vi "Test Bench v13 - TDMS.vi"() -> ()   [LabVIEW 2022 SP3]
uses:
  WhiteNoise.ctl
  <vilib>/Utility/error.llb/DialogType.ctl
  <vilib>/DAQmx/read.llb/DAQmx Read (Analog 1D DBL 1Chan NSamp).vi
  <vilib>/DAQmx/write.llb/DAQmx Write (Analog 2D DBL NChan NSamp).vi
  <vilib>/DAQmx/create/channels.llb/DAQmx Create Channel (AI-Acceleration-Accelerometer).vi
  <vilib>/DAQmx/create/channels.llb/DAQmx Create Channel (AO-Voltage-Basic).vi
  <vilib>/DAQmx/configure/timing.llb/DAQmx Timing (Sample Clock).vi
  <vilib>/DAQmx/miscellaneous.llb/DAQmx Fill In Error Info.vi
  <resource>/objmgr/daqmx.rc
  <vilib>/measure/NI_MABase.lvlib
panel:
  in  "Enable Display":bool=TRUE
  in  "Folder to save file to":path=path "C:/Users/LAV-UFSC/OneDrive - UFSC/Documents-LAV-UFSC/LAV-TCC/Dados-Experimentos/Dados-Bancada-LABVIEW"
  out "Waveform Chart 3":dbl[](graph)
  out "Waveform Chart":dynamicdata(graph)
  in  "Accel. 2":bool
  in  "Start\nReading":bool=TRUE
  out "New file path":path
  in  "Signal Output\nControl":enum32{"White Noise", "Harmonic"}(tab)
  in  "White Noise\nParameters":T2={"Seed"=0.0, "Standard Deviation"=0.2, "Reset"=FALSE, "Iterator"=1.0, "Seed"=-1, "Stop 4"=FALSE, "Lower Cut-Off"=5.0, "Upper Cut-Off"=350.0} {"Upper Cut-Off" min=5.0 max=350.0 step=10.0; "Lower Cut-Off" min=5.0 max=350.0 step=10.0; "Standard Deviation" min=0.001 max=1.5 step=0.05 format="%0.2p"}
  out "dt White Noise":dbl
  in  "Hamonic\nParameters":T3={"Waveform Type"=0, "Frequency"=10.0, "Amplitude"=0.25, "Stop 4"=FALSE} {"Frequency" min=5.0 max=350.0 step=10.0 format="%0.2p"; "Waveform Type" items=["Sine Wave", "Triangle Wave", "Square Wave", "Sawtooth Wave"]; "Amplitude" min=0.001 max=0.3 step=0.05 format="%0.2p"}
  out "dt Harmonic":dbl
  in  "Start\nOutput":bool=TRUE
  # "Filter"
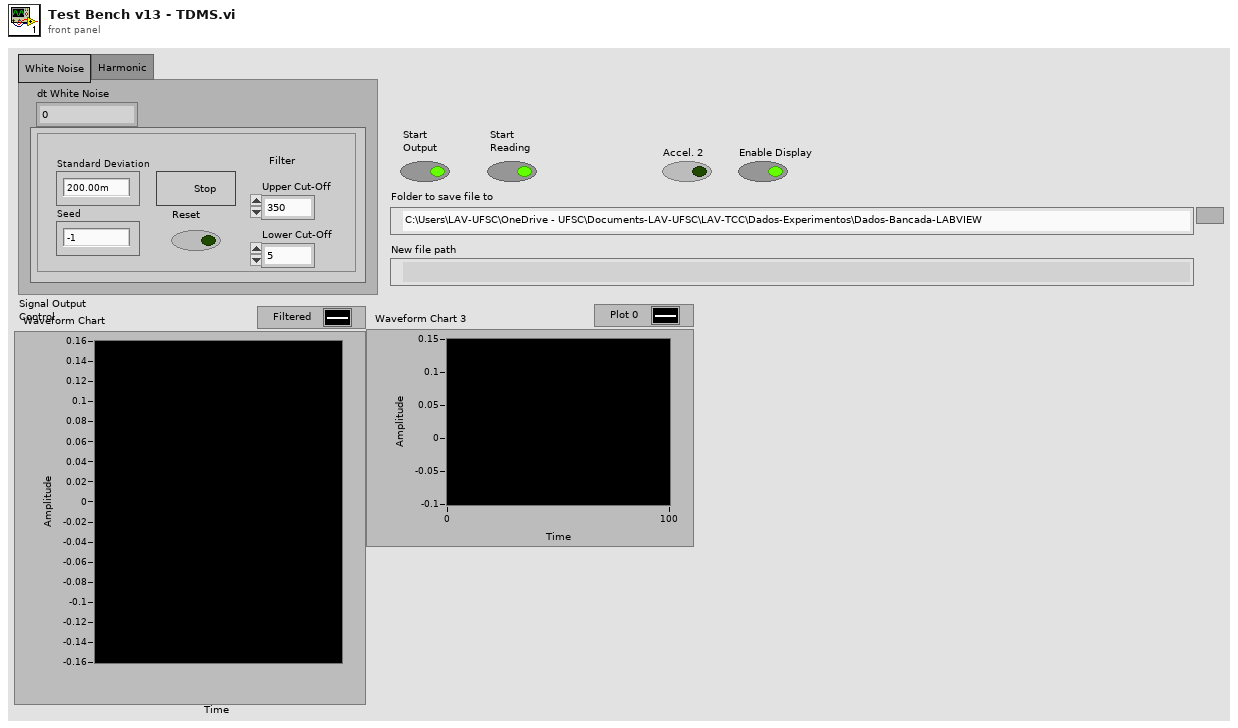
[diagram p1: front panel]
types:
  T1 = typedef "WhiteNoise.ctl" = dbl
  T2 = cluster{"Seed":T1, "Standard Deviation":dbl, "Reset":bool, "Iterator":dbl, "Seed":i8, "Stop 4":bool, "Lower Cut-Off":dbl, "Upper Cut-Off":dbl}
  T3 = cluster{"Waveform Type":u16, "Frequency":dbl, "Amplitude":dbl, "Stop 4":bool}
  T4 = enum16{"open", "open or create", "create or replace", "create", "open (read-only)"}
  T5 = typedef "DialogType.ctl" = u16
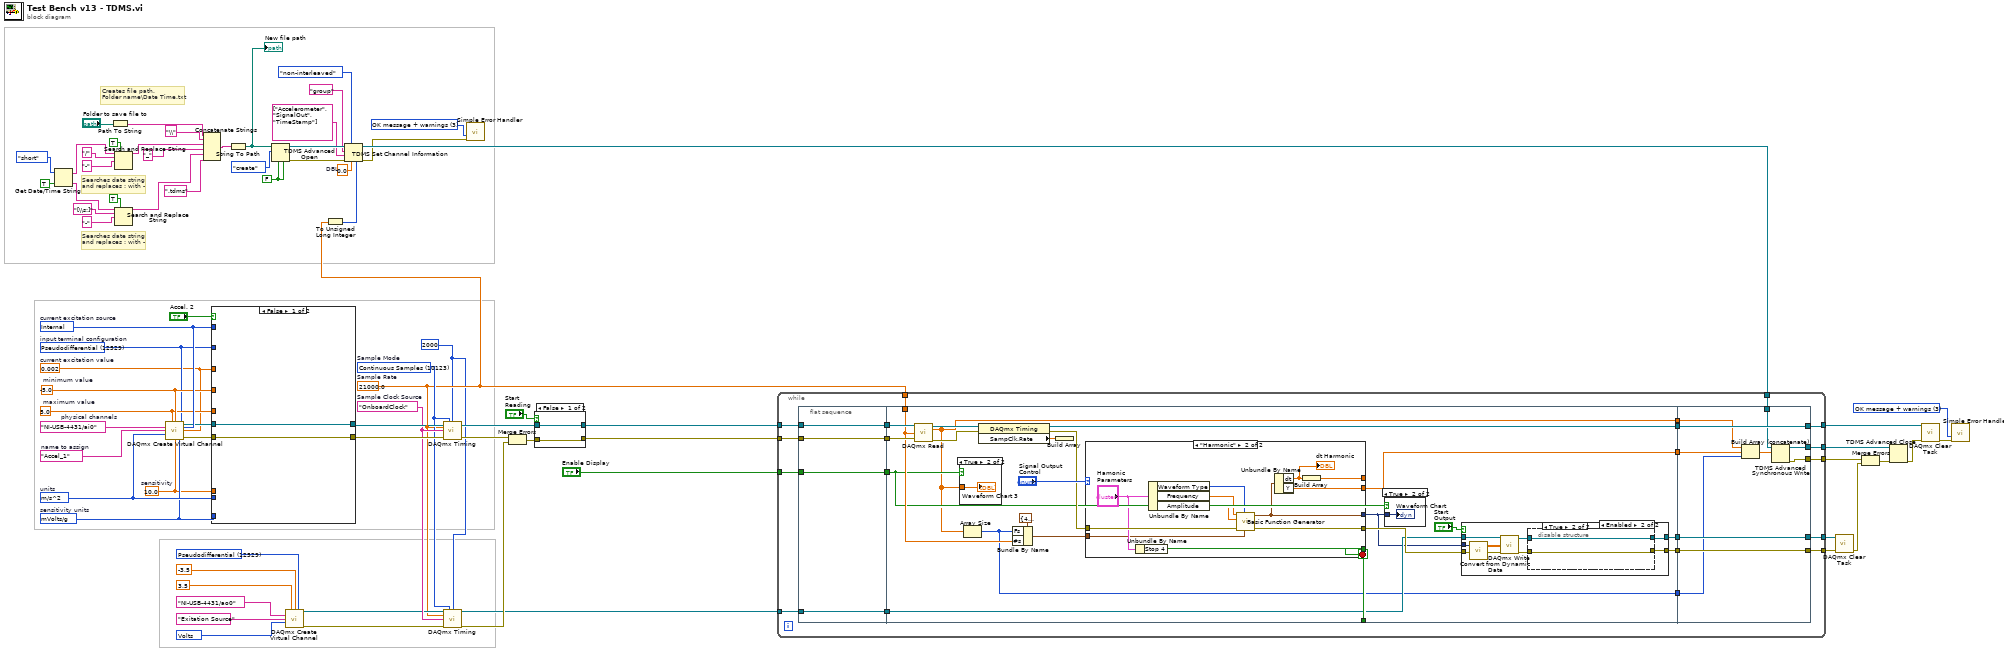
[diagram p0: block diagram]
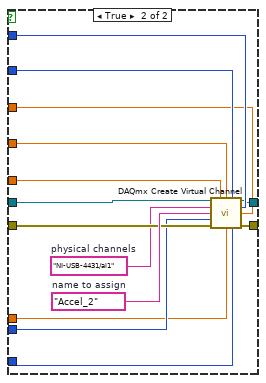
[diagram p2: hidden frame]
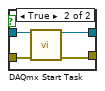
[diagram p3: hidden frame]
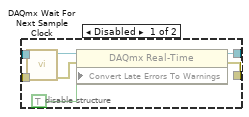
[diagram p7: hidden frame]
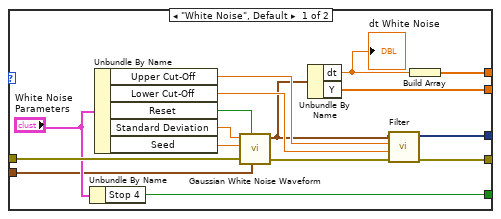
[diagram p8: hidden frame]
diagram:
  w1 = 2000 ("samples per channel")
  w9 = 0.0  # DBL
  w11 = FALSE ("enable asynchronous? (T)")
  w7 = T5 3 items=["no dialog", "OK message", "continue or stop message", "OK message + warnings", "continue/stop + warnings"] ("type of dialog (OK msg:1)")
  w54 = T5 3 items=["no dialog", "OK message", "continue or stop message", "OK message + warnings", "continue/stop + warnings"] ("type of dialog (OK msg:1)")
  w64 = 12529 items=["Default"=-1, "RSE"=10083, "Differential"=10106, "Pseudodifferential"=12529] ("output terminal configuration")
  w62 = 10348 items=["Volts"=10348, "From Custom Scale"=10065] ("units")
  w68 = 12509 items=["mVolts/g"=12509, "Volts/g"=12510]  # sensitivity units
  w58 = 10.0  # sensitivity
  w67 = 0.002  # current excitation value
  w75 = 10200 items=["Internal"=10200, "External"=10167, "None"=10230]  # current excitation source
  w69 = tag "NI-USB-4431/ai0"  # physical channels
  w55 = tag "OnboardClock"  # Sample Clock Source
  w5 = 21000.0  # Sample Rate
  w53 = 10123 items=["Finite Samples"=10178, "Continuous Samples"=10123, "Hardware Timed Single Point"=12522]  # Sample Mode
  w71 = 12529 items=["default"=-1, "RSE"=10083, "NRSE"=10078, "Differential"=10106, "Pseudodifferential"=12529]  # input terminal configuration
  w74 = -5.0  # minimum value
  w73 = 5.0  # maximum value
  w77 = "Accel_1"  # name to assign
  w72 = 12470 items=["g"=10186, "m/s^2"=12470, "in/s^2"=12471, "From Custom Scale"=10065]  # units
  # "Searches date string\nand replaces : with -"
  # "Searches date string\nand replaces : with -"
  # "Creates file path.\nFolder name\\Date Time.txt"
  n1 = Get Date/Time String(date format (0)=enum16{"short", "long", "abbreviated"}."short", want seconds? (F)=TRUE) -> (date string=w20:string, time string=w34:string)  [unwired: 1 in]
  n2 = Path To String(path="Folder to save file to") -> (string=w28:string)
  n3 = Search and Replace String(replace all?=TRUE ("replace all? (F)"), input string=w20, search string="/" ("replace string (\"\")"), replace string="-" ("replace string (\"\")")) -> (result string=w19:string)  [unwired: 4 in, 3 out]
  n4 = Search and Replace String(replace all?=TRUE ("replace all? (F)"), input string=w34, search string="[\\s:]" ("replace string (\"\")"), replace string="-" ("replace string (\"\")")) -> (result string=w26:string)  [unwired: 4 in, 3 out]
  n5 = call-poly <vilib>:"DAQmx Create Virtual Channel.vi"("maximum value"=w73, "minimum value"=w74, "input terminal configuration"=w71, "physical channels"=w69, "current excitation source"=w75, "name to assign"=w77, "current excitation value"=w67, "units"=w72, "sensitivity"=w58, "sensitivity units"=w68) -> ("task out"=w70:refnum<k21>, "error out"=w76:errorcluster)  [unwired: 4 in]
  n6 = Concatenate Strings(w28, "\\" ("string"), w19, "_" ("string"), w26, ".tdms" ("string")) -> (w24:string)
  n7 = case shown="False" "Accel. 2" {
    tunnel: w76 -> [w79 w92]
    tunnel: w75 -> [_ w91]
    tunnel: w74 -> [_ w90]
    tunnel: w73 -> [_ w89]
    tunnel: w72 -> [_ w88]
    tunnel: w71 -> [_ w87]
    tunnel: w70 -> [w78 w86]
    tunnel: w68 -> [_ w84]
    tunnel: w67 -> [_ w83]
    tunnel: w58 -> [_ w82]
    tunnel: [w79 w81] -> w57
    tunnel: [w78 w80] -> w56
    frame False {
    }
    frame True {
      w85 = tag "NI-USB-4431/ai1"  # physical channels
      w93 = "Accel_2"  # name to assign
      n8 = call-poly <vilib>:"DAQmx Create Virtual Channel.vi"("task in"=w86, "maximum value"=w89, "minimum value"=w90, "input terminal configuration"=w87, "physical channels"=w85, "current excitation source"=w91, "name to assign"=w93, "current excitation value"=w83, "units"=w88, "error in"=w92, "sensitivity"=w82, "sensitivity units"=w84) -> ("task out"=w80:refnum<k21>, "error out"=w81:errorcluster)  [unwired: 2 in]
    }
  }
  n9 = String To Path(string=w24) -> (path=w39:path)
  "New file path" <- w39
  n10 = TDMS Advanced Open(4:w11, 6:w11, 10:T4."create" ("operation (0:open)"), 11:w39) -> (0:w15:errorcluster, 3:w14:refnum<k34>)  [unwired: 1 in, 1 out]
  n11 = call-poly <vilib>:"DAQmx Create Virtual Channel.vi"("maximum value"=3.5, "minimum value"=-3.5, "output terminal configuration"=w64, "physical channels"=tag "NI-USB-4431/ao0", "name to assign"="Exitation Source", "units"=w62) -> ("task out"=w51:refnum<k21>, "error out"=w52:errorcluster)  [unwired: 8 in]
  n12 = To Unsigned Long Integer(number=w5) -> (unsigned 32bit integer=w6:u32)
  n13 = TDMS Set Channel Information(4:w6, 6:w9, 7:enum16{"non-interleaved", "interleaved"}."non-interleaved" ("data layout (0:non-interleaved)"), 8:w15, 9:string[] ["Accelerometer", "SignalOut", "TimeStamp"] ("channel name(s)"), 10:"group" ("group name (Untitled)"), 11:w14) -> (0:w8:errorcluster, 3:w38:refnum<k34>)
  n14 = call-poly <vilib>:"DAQmx Timing.vi"("task/channels in"=w56, "sample mode"=w53, "samples per channel"=w1, "rate"=w5, "source"=w55, "error in"=w57) -> ("task out"=w60:refnum<k21>, "error out"=w61:errorcluster)  [unwired: 8 in]
  n15 = call-poly <vilib>:"DAQmx Timing.vi"("task/channels in"=w51, "sample mode"=w53, "samples per channel"=w1, "rate"=w5, "source"=w55, "error in"=w52) -> ("task out"=w49:refnum<k21>, "error out"=w50:errorcluster)  [unwired: 8 in]
  n16 = call <vilib>:"Simple Error Handler.vi"("type of dialog (OK msg:1)"=w7, "error in (no error)"=w8) -> ()  [unwired: 3 in, 5 out]
  n17 = Merge Errors(w61, w50) -> (w42:errorcluster)
  n18 = case shown="False" "Start\nReading" {
    tunnel: [w94 w96] -> w44
    tunnel: [w95 w97] -> w43
    tunnel: w42 -> [w95 w98]
    tunnel: w60 -> [w94 w99]
    frame False {
    }
    frame True {
      n19 = call <vilib>:"DAQmx Start Task.vi"("task/channels in"=w99, "error in"=w98) -> ("task out"=w96:refnum<k21>, "error out"=w97:errorcluster)  [unwired: 12 in]
    }
  }
  n20 = while {
    tunnel: w49 -> [w121]
    tunnel: [w117] -> w48
    tunnel: [w118] -> w47
    tunnel: w44 -> [w120]
    tunnel: w43 -> [w119]
    tunnel: [w115] -> w40
    tunnel: w38 -> [w105]
    tunnel: [w103] -> w37
    tunnel: w5 -> [w114]
    tunnel: "Enable Display" -> [w113]
    tunnel: [w104] -> w3
    stop <- w116 stop-if-true
    n21 = flat-sequence {
      tunnel: w113 -> [w122]
      tunnel: w119 -> [w123]
      tunnel: w120 -> [w124]
      tunnel: w121 -> [w125]
      tunnel: [w125] -> w112
      tunnel: [w124] -> w111
      tunnel: [w123] -> w110
      tunnel: [w122] -> w109
      tunnel: [w140] -> w116
      tunnel: w114 -> [w133]
      tunnel: w112 -> [w145]
      tunnel: w111 -> [w144]
      tunnel: w110 -> [w143]
      tunnel: w109 -> [w129]
      tunnel: [w142] -> w108
      tunnel: [w141] -> w107
      tunnel: [w137] -> w106
      tunnel: [w128] -> w102
      tunnel: [w127] -> w101
      tunnel: [w126] -> w100
      tunnel: [w204] -> w115
      tunnel: [w205] -> w117
      tunnel: [w206] -> w118
      tunnel: w108 -> [w206]
      tunnel: w107 -> [w205]
      tunnel: w106 -> [w204]
      tunnel: w105 -> [w203]
      tunnel: [w202] -> w104
      tunnel: [w201] -> w103
      tunnel: w102 -> [w199]
      tunnel: w101 -> [w198]
      tunnel: w100 -> [w197]
      frame #0 {
      }
      frame #1 {
        n22 = call-poly <vilib>:"DAQmx Read.vi"("task/channels in"=w144, "number of samples per channel"=w133, "error in"=w143) -> ("task out"=w138:refnum<k21>, "data"=w128:dbl[], "error out"=w136:errorcluster)  [unwired: 10 in]
        n23 = case shown="True" w129 {
          tunnel: w128 -> [_ w148]
          frame False {
          }
          frame True {
            "Waveform Chart 3" <- w148
          }
        }
        n24 = Array Size(array=w128) -> (size(s)=w126:i32)
        n25 = property class="DAQmx Timing"(reference=w138, error in=w136) -> (reference out=w137:refnum<k21>, error out=w135:errorcluster, "SampClk.Rate"=w131:dbl)
        n26 = Bundle By Name(cluster=cluster{"Fs":dbl, "#s":dbl} {"Fs"=41200.0, "#s"=41200.0} ("sampling info"), "Fs"=w126, "#s"=w133) -> (w134:cluster{"Fs":dbl, "#s":dbl})
        n27 = Build Array(w131) -> ()  [unwired: 1 out]
        n28 = case shown="\"Harmonic\"" "Signal Output\nControl" {
          tunnel: w135 -> [w184 w196]
          tunnel: [w181 w195] -> w146
          tunnel: [w183 w193] -> w140
          tunnel: w134 -> [w179 w192]
          tunnel: [w171 w187] -> _
          tunnel: [w170 w186] -> w130
          tunnel: [w169 w185] -> w127
          frame "White Noise", Default {
            n29 = Unbundle By Name("White Noise\nParameters") -> ("Stop 4"=w183:bool)
            n30 = Unbundle By Name("White Noise\nParameters") -> ("Upper Cut-Off"=w175:dbl, "Lower Cut-Off"=w174:dbl, "Reset"=w176:bool, "Standard Deviation"=w177:dbl, "Seed"=w178:T1)
            n31 = call <vilib>:"Gaussian White Noise Waveform.vi"("sampling info"=w179, "reset signal"=w176, "error in (no error)"=w184, "seed"=w178, "standard deviation"=w177) -> ("error out"=w182:errorcluster, "signal out"=w173:waveform(dbl))  [unwired: 5 in]
            n32 = Unbundle By Name(w173) -> ("dt"=w172:dbl, "Y"=w169:dbl[])
            "dt White Noise" <- w172
            n33 = call "Filter"("error in (no error)"=w182, "Lower Cut-Off"=w174, "Upper Cut-Off"=w175, "Signal"=w173) -> ("error out"=w181:errorcluster, "Filtered Signal"=w170:dynamicdata)  [unwired: 6 in]
            n34 = Build Array(w172) -> (w171:dbl[])
          }
          frame "Harmonic" {
            n35 = Unbundle By Name("Hamonic\nParameters") -> ("Stop 4"=w193:bool)
            n36 = Unbundle By Name("Hamonic\nParameters") -> ("Waveform Type"=w191:u16, "Frequency"=w190:dbl, "Amplitude"=w189:dbl)
            n37 = call <vilib>:"Basic Function Generator.vi"("sampling info"=w192, "signal type"=w191, "error in (no error)"=w196, "amplitude"=w189, "frequency"=w190) -> ("error out"=w195:errorcluster, "signal out"=w186:waveform(dbl))  [unwired: 4 in, 1 out]
            n38 = Unbundle By Name(w186) -> ("dt"=w188:dbl, "Y"=w185:dbl[])
            "dt Harmonic" <- w188
            n39 = Build Array(w188) -> (w187:dbl[])
          }
        }
        n40 = case shown="True" w129 {
          tunnel: w130 -> [_ w149]
          frame False {
          }
          frame True {
            "Waveform Chart" <- w149
          }
        }
        n41 = case shown="True" "Start\nOutput" {
          tunnel: w146 -> [w150 w159]
          tunnel: w145 -> [w151 w158]
          tunnel: [w150 w154] -> w142
          tunnel: [w151 w155] -> w141
          tunnel: w130 -> [_ w153]
          frame False {
          }
          frame True {
            n42 = call "Convert from Dynamic Data"("Dynamic Data Type"=w153) -> ("Array"=w152:dbl[][])  [unwired: 3 in]
            n43 = call-poly <vilib>:"DAQmx Write.vi"("task/channels in"=w158, "data"=w152, "error in"=w159) -> ("task out"=w157:refnum<k21>, "error out"=w156:errorcluster)  [unwired: 10 in, 1 out]
            n44 = disable-structure shown="Enabled" {
              disable-tunnel: w157 -> [w166 w167]
              disable-tunnel: w156 -> [w165 w168]
              disable-tunnel: [w163 w167] -> w155
              disable-tunnel: [w162 w168] -> w154
              frame Disabled {
                n45 = call <vilib>:"DAQmx Wait For Next Sample Clock.vi"("task/channels in"=w166, "error in"=w165) -> ("task out"=w164:refnum<k21>, "error out"=w161:errorcluster)  [unwired: 11 in, 1 out]
                n46 = property class="DAQmx Real-Time"(reference=w164, error in=w161, "Convert Late Errors To Warnings"=TRUE ("ConvLateErrorsToWarnings")) -> (reference out=w163:refnum<k21>, error out=w162:errorcluster)
              }
              frame Enabled {
              }
            }
          }
        }
      }
      frame #2 {
        n47 = Build Array (concatenate)(w199, w198, w197) -> (w200:dbl[])
        n48 = TDMS Advanced Synchronous Write(10:w200, 11:w203) -> (0:w202:errorcluster, 3:w201:refnum<k34>)  [unwired: 1 in]
      }
    }
  }
  n49 = call <vilib>:"DAQmx Clear Task.vi"("task in"=w48, "error in"=w47) -> ("error out"=w2:errorcluster)  [unwired: 13 in]
  n50 = Merge Errors(w3, w2) -> (w4:errorcluster)
  n51 = TDMS Advanced Close(8:w4, 11:w37) -> (0:w17:errorcluster)  [unwired: 2 in, 1 out]
  n52 = call <vilib>:"DAQmx Clear Task.vi"("task in"=w40, "error in"=w17) -> ("error out"=w41:errorcluster)  [unwired: 13 in]
  n53 = call <vilib>:"Simple Error Handler.vi"("type of dialog (OK msg:1)"=w54, "error in (no error)"=w41) -> ()  [unwired: 3 in, 5 out]
